vi "fgv_graphbase-slam_edge.vi"(7 "cmd":T3, 11 "pf-val":T2={"Q"=[[0.04000000000000001]], "Q_sim"=[[0.04000000000000001]], "d1"=0.0, "d2"=0.0, "yaw1"=0.0, "yaw2"=0.0, "angle1"=0.0, "angle2"=0.0, "id1"=0, "id2"=0}) -> (3 "pf-val out":T2={"Q"=[[0.04000000000000001]], "Q_sim"=[[0.04000000000000001]], "d1"=0.0, "d2"=0.0, "yaw1"=0.0, "yaw2"=0.0, "angle1"=0.0, "angle2"=0.0, "id1"=0, "id2"=0})   [LabVIEW 2019]
uses:
  Ctrl/cmd_common.ctl
  <vilib>/Analysis/Matrix/Datatypes/RealMatrix.ctl
  <vilib>/Analysis/Matrix/NI_Matrix.lvlib
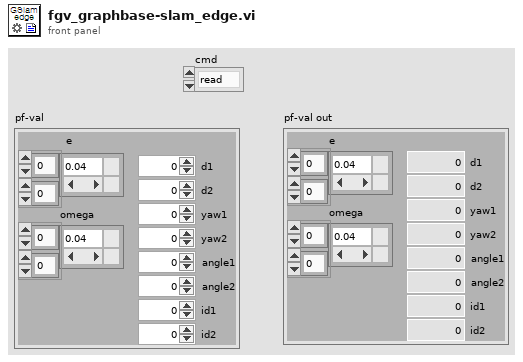
[diagram p1: front panel]
types:
  T1 = typedef "NI_Matrix.lvlib/RealMatrix.ctl" = dbl[][]
  T2 = cluster{"Q":T1, "Q_sim":T1, "d1":dbl, "d2":dbl, "yaw1":dbl, "yaw2":dbl, "angle1":dbl, "angle2":dbl, "id1":u32, "id2":u32}
  T3 = typedef "cmd_common.ctl" = enum16{"read", "write"}
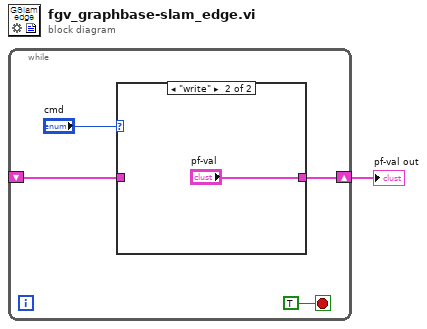
[diagram p0: block diagram]
diagram:
  n1 = while {
    shift-right: [w3] -> w1
    shift-left: _ -> [w2]
    stop <- TRUE stop-if-true
    n2 = case shown="\"write\"" "cmd" {
      tunnel: [w6 "pf-val"] -> w3
      tunnel: w2 -> [w6 _]
      frame "read", Default {
      }
      frame "write" {
      }
    }
  }
  "pf-val out" <- w1
